vi "Plot Global.vi"() -> ()   [LabVIEW 2016]
panel:
  in  "Type":T1(ring)
  out "Data":variant
  in  "Dimensions":u8
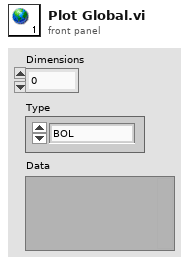
[diagram p1: front panel]
types:
  T1 = enum8{"BOL", "U8", "U16", "U32", "U64", "I8", "I16", "I32", "I64", "SGL", "DBL", "EXT", "CSG", "CDB", "CXT", "STR", "TBL", "TLU", "CTM"}
diagram:
